vi "write engine configuration.vi"(8 "error in":errorcluster, 10 "engine configuration":refnum<class "engine configuration.lvclass">, 11 "Engine Parent Editor Node in":refnum<class "Engine Parent Editor Node.lvclass">) -> (0 "error out":errorcluster, 3 "Engine Parent Editor Node out":refnum<class "Engine Parent Editor Node.lvclass">)   [LabVIEW 2013, in "PL Framework Configuration Tool.lvlib" / "Engine Parent Editor Node.lvclass"]
uses:
  Engine Parent Editor Node.lvclass
  <vilib>/NI/Module Execution Interface/Engine Configuration/engine configuration.lvclass
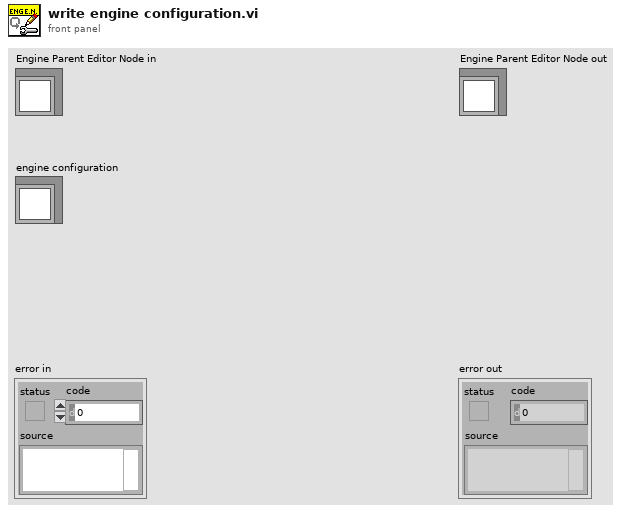
[diagram p1: front panel]
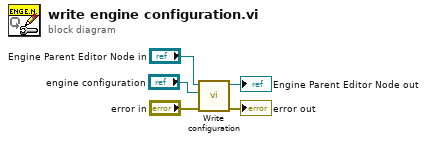
[diagram p0: block diagram]
diagram:
  n1 = call-dynamic "Write configuration.vi"("error in"="error in", "configuration"="engine configuration", "NISE_CEF_serializable node in"="Engine Parent Editor Node in") -> ("error out"=→"error out":errorcluster, "NISE_CEF_serializable node out"=→"Engine Parent Editor Node out":refnum<class "Engine Parent Editor Node.lvclass">)  [unwired: 7 in]
